vi "Execution Abort.vi"(8 "error in (no error)":errorcluster, 11 "teststand-api in":refnum<class "teststand-api.lvclass">) -> (0 "error out":errorcluster, 3 "teststand-api out":refnum<class "teststand-api.lvclass">)   [LabVIEW 2014, in "teststand-api.lvlib" / "teststand-api.lvclass"]
uses:
  teststand-api.lvclass
  teststand-api.lvclass/teststand-api.ctl
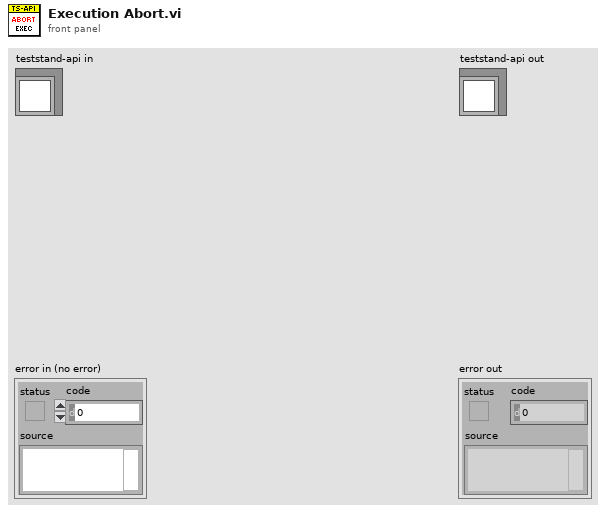
[diagram p1: front panel]
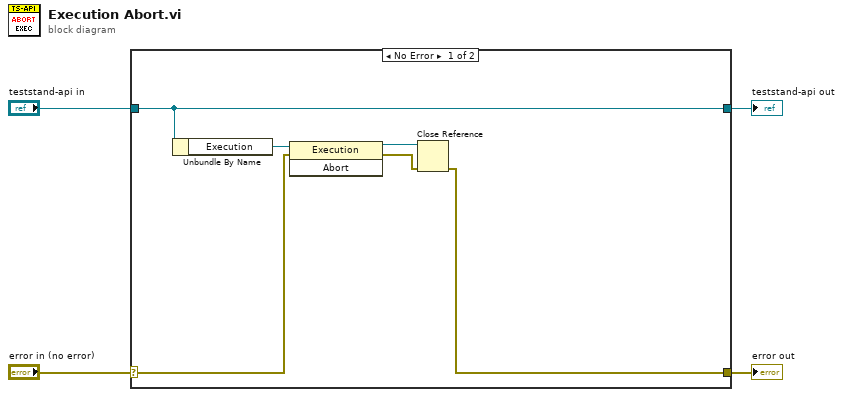
[diagram p0: block diagram]
diagram:
  n1 = case shown="No Error" "error in (no error)" {
    selector: "error in (no error)" -> [w8 w12]
    tunnel: [w5 w12] -> w3
    tunnel: [w10 w11] -> w1
    tunnel: "teststand-api in" -> [w10 w11]
    frame No Error {
      n2 = Unbundle By Name(w10) -> ("Execution"=w9:refnum<k7>)
      n3 = invoke class="Execution" method="Abort"(reference=w9, error in=w8) -> (reference out=w7:refnum<k7>, error out=w6:errorcluster)  [unwired: 1 in, 1 out]
      n4 = Close Reference(reference=w7, error in (no error)=w6) -> (error out=w5:errorcluster)
    }
    frame Error {
    }
  }
  "error out" <- w3
  "teststand-api out" <- w1
